vi "pack frame.vi"(4 "switch bitrate? (F)":bool, 6 "can fd? (F)":bool, 7 "extended id?":bool, 8 "remote transmission request? (F)":bool, 10 "data":u8[](array[numeric]) format="%x", 11 "id":u32 format="%x") -> (3 "frame":u8[](array[numeric]) format="%x")   [LabVIEW 2024, in "atsj peakcan basic.lvlib"]
uses:
  atsj peakcan basic.lvlib
  message type.ctl
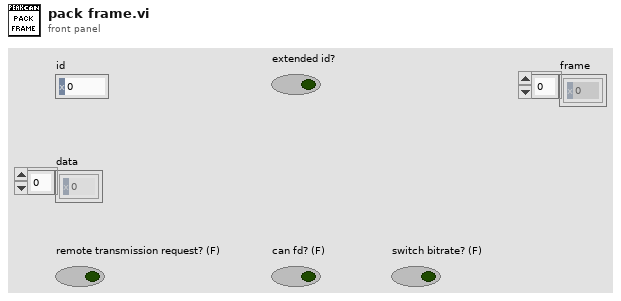
[diagram p1: front panel]
types:
  T1 = typedef "atsj peakcan basic.lvlib/message type.ctl" = cluster{"standard":bool, "remote transmission request ":bool, "extended":bool, "fd":bool, "fd bit rate switch":bool, "fd error state":bool, "echo":bool, "error":bool, "status":bool}
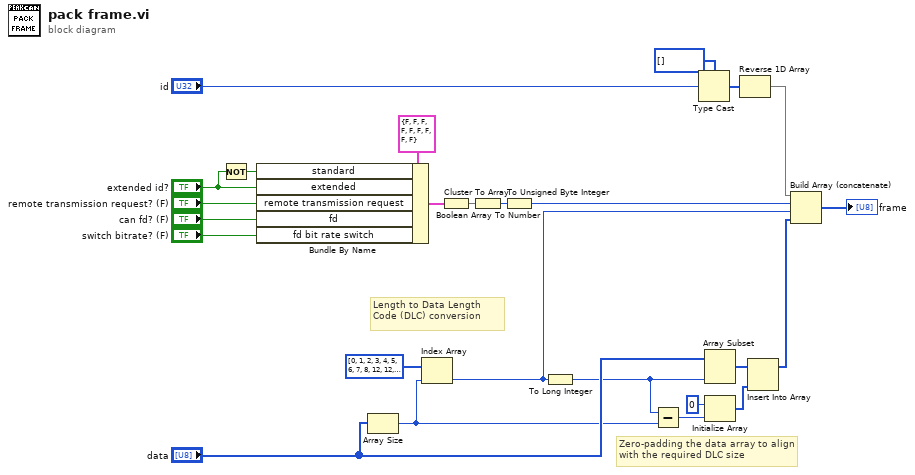
[diagram p0: block diagram]
diagram:
  # "Zero-padding the data array to align with the required DLC size"
  # "Length to Data Length Code (DLC) conversion"
  n1 = Not(x="extended id?") -> (.not. x?=w1:bool)
  n2 = Bundle By Name(cluster=T1 {"standard"=FALSE, "remote transmission request "=FALSE, "extended"=FALSE, "fd"=FALSE, "fd bit rate switch"=FALSE, "fd error state"=FALSE, "echo"=FALSE, "error"=FALSE, "status"=FALSE}, "standard"=w1, "extended"="extended id?", "remote transmission request"="remote transmission request? (F)", "fd"="can fd? (F)", "fd bit rate switch"="switch bitrate? (F)") -> (w3:T1)
  n3 = Array Size(array="data") -> (size(s)=w17:i32)
  n4 = Index Array(array=u8[] [0, 1, 2, 3, 4, 5, 6, 7, 8, 12, 12, 12, 12, 16, 16, 16, 16, 20, 20, 20, 20, 24, 24, 24, 24, 32, 32, 32, 32, 32, 32, 32, 32, 48, 48, 48, 48, 48, 48, 48, 48, 48, 48, 48, 48, 48, 48, 48, 48, 64, 64, 64, 64, 64, 64, 64, 64, 64, 64, 64, 64, 64, 64, 64, 64] ("Array"), index=w17) -> (element=w18:u8)
  n5 = Cluster To Array(cluster=w3) -> (array=w6:bool[])
  n6 = Boolean Array To Number(Boolean array=w6) -> (number=w7:u32)
  n7 = To Unsigned Byte Integer(number=w7) -> (unsigned 8bit integer=w10:u8)
  n8 = To Long Integer(number=w18) -> (32bit integer=w19:i32)
  n9 = Subtract(x=w19, y=w17) -> (x-y=w14:i32)
  n10 = Type Cast(type=u8[] [], x="id") -> (*(type *) &x=w9:u8[])
  n11 = Array Subset(array="data", length=w19) -> (w15:u8[])  [unwired: 1 in]
  n12 = Initialize Array(u8 0, w14) -> (w16:u8[])
  n13 = Reverse 1D Array(array=w9) -> (reversed array=w11:u8[])
  n14 = Insert Into Array(array=w15, new element=w16) -> (w20:u8[])  [unwired: 1 in]
  n15 = Build Array (concatenate)(w11, w10, w18, w20) -> (→"frame":u8[])
